vi "Shutdown All.vi"(8 "error in (no error)":errorcluster, 11 "Thread Manager in":refnum<class "Thread Manager.lvclass">) -> (0 "error out":errorcluster, 3 "Thread Manager out":refnum<class "Thread Manager.lvclass">)   [LabVIEW 2019, in "DSF Core.lvlib" / "Thread Manager.lvclass"]
uses:
  Thread Manager.lvclass
  Thread Manager.lvclass/Thread Manager.ctl
  Thread/Thread.lvclass
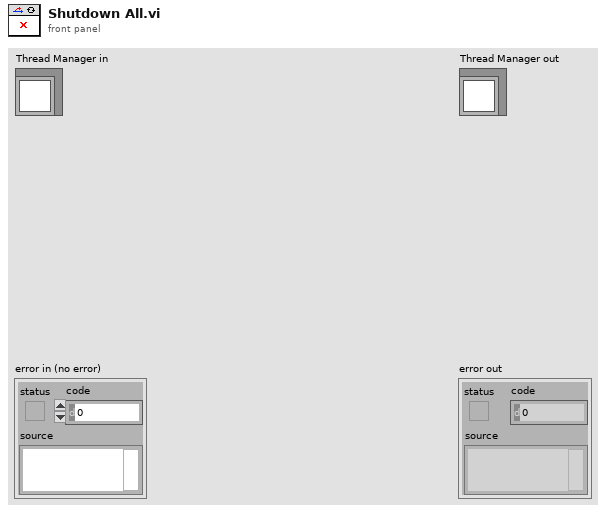
[diagram p1: front panel]
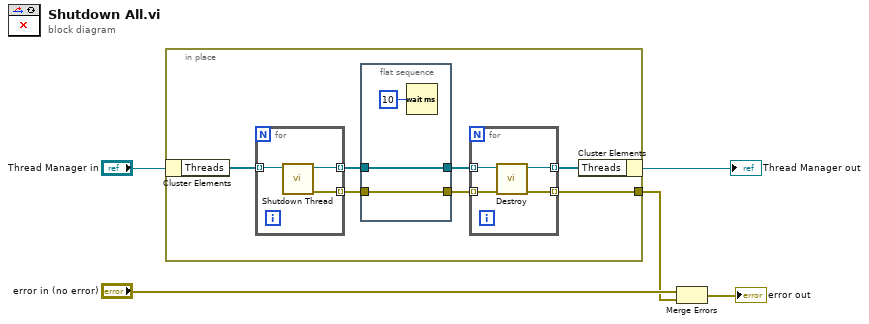
[diagram p0: block diagram]
diagram:
  n1 = in-place {
    in-place-border: [w11] -> w1
    n2 = in-place-cluster #1("Thread Manager in") -> ("Threads"=w12:refnum<class "Thread.lvclass">[])
    n3 = for {
      tunnel: w12 -> [w22] mode=indexing
      tunnel: [w21] -> w9 mode=indexing
      tunnel: [w20] -> w8 mode=indexing
      n4 = call "Shutdown Thread.vi"("Thread in"=w22) -> ("error out"=w20:errorcluster, "Thread out"=w21:refnum<class "Thread.lvclass">)  [unwired: 9 in]
    }
    n5 = flat-sequence {
      tunnel: w9 -> [w15]
      tunnel: w8 -> [w14]
      tunnel: [w15] -> w7
      tunnel: [w14] -> w6
      frame #0 {
        n6 = Wait (ms)(milliseconds to wait=u32 10) -> ()  [unwired: 1 out]
      }
    }
    n7 = for {
      tunnel: w7 -> [w19] mode=indexing
      tunnel: [w18] -> w10 mode=indexing
      tunnel: [w17] -> w11 mode=indexing
      tunnel: w6 -> [w16] mode=indexing
      n8 = call-dynamic "Destroy.vi"("error in (no error)"=w16, "Thread"=w19) -> ("error out"=w17:errorcluster, "Thread type"=w18:refnum<class "Thread.lvclass">)  [unwired: 8 in]
    }
    n9 = in-place-cluster #1("Threads"=w10) -> (→"Thread Manager out":refnum<class "Thread Manager.lvclass">)
  }
  n10 = Merge Errors("error in (no error)", w1) -> (→"error out":errorcluster)
